vi "Write String.vi"(8 "error in":errorcluster, 10 "Value":string, 11 "String Control Reference in":refnum<vi>) -> (0 "error out":errorcluster, 3 "String Control Reference out":refnum<vi>)   [LabVIEW 2020, in "G-Unicode.lvlib"]
uses:
  G-Unicode.lvlib
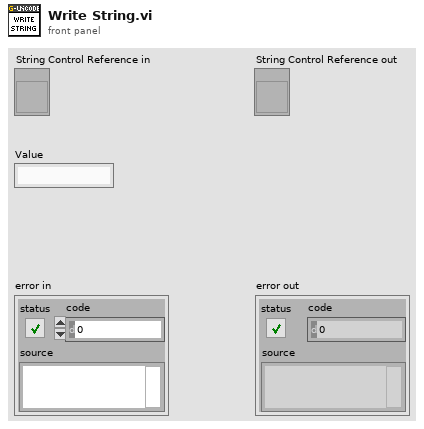
[diagram p1: front panel]
types:
  T1 = cluster{"Text.Selection End":u32, "Text.Selection End":u32}
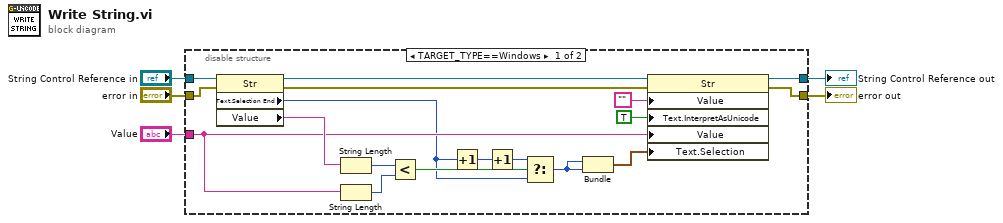
[diagram p0: block diagram]
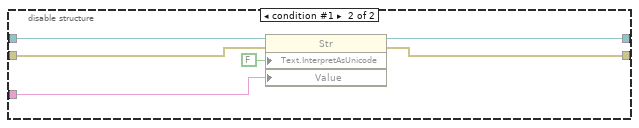
[diagram p2: hidden frame]
diagram:
  n1 = disable-structure shown="TARGET_TYPE==Windows" {
    disable-tunnel: [w23 w29] -> w5
    disable-tunnel: [w22 w28] -> w4
    disable-tunnel: "String Control Reference in" -> [w19 w27]
    disable-tunnel: "error in" -> [w17 w25]
    disable-tunnel: "Value" -> [w14 w26]
    frame condition #0 (active) {
      n2 = property class="Str"(reference=w19, error in=w17) -> (reference out=w18:refnum<vi>, error out=w16:errorcluster, "Text.Selection End"=w6:u32, "Value"=w15:string)
      n3 = String Length(string=w15) -> (length=w13:i32)
      n4 = String Length(string=w14) -> (length=w12:i32)
      n5 = Less?(x=w13, y=w12) -> (x < y?=w11:bool)
      n6 = Increment(x=w6) -> (x+1=w9:u32)
      n7 = Increment(x=w9) -> (x+1=w7:u32)
      n8 = Select(t=w7, s=w11, f=w6) -> (s? t:f=w10:u32)
      n9 = Bundle("Text.Selection End"=w10, "Text.Selection End"=w10) -> (w8:T1)  [unwired: 1 in]
      n10 = property class="Str"(reference=w18, error in=w16, "Value"="", "Text.InterpretAsUnicode"=TRUE ("Text.Interpret As Unicode"), "Value"=w14, "Text.Selection"=w8) -> (reference out=w23:refnum<vi>, error out=w22:errorcluster)
    }
    frame condition #1 {
      n11 = property class="Str"(reference=w27, error in=w25, "Text.InterpretAsUnicode"=FALSE ("Text.Interpret As Unicode"), "Value"=w26) -> (reference out=w29:refnum<vi>, error out=w28:errorcluster)
    }
  }
  "String Control Reference out" <- w5
  "error out" <- w4
